vi "Ejemplo Vehiculo Motor.vi"   [LabVIEW 2020]
uses:
  Vehiculo Motor/Vehiculo de Motor.lvclass
  Vehiculo Motor/Write Tipo Motor.vi
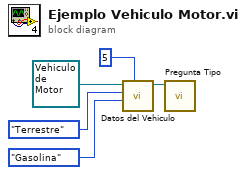
[diagram p0: block diagram]
diagram:
  n1 = call "Datos del Vehiculo.vi"("#Pasajeros"=u16 5, "Tipo Motor"=enum16{"Eléctrico", "Gasolina"}."Gasolina", "Ambiente de operacion"=enum16{"Acuático", "Terrestre", "Aereo"}."Terrestre", "Vehiculo de Motor in"=refnum<class "Vehiculo de Motor.lvclass"> refnum ("Vehiculo de Motor.lvclass")) -> ("Vehiculo de Motor out"=w1:refnum<class "Vehiculo de Motor.lvclass">)  [unwired: 6 in, 1 out]
  n2 = call "Pregunta Tipo.vi"("Vehiculo de Motor in"=w1) -> ()  [unwired: 9 in, 2 out]
